vi "Slave - Interleaved Chs Dat Integrity.vi"() -> ()   [LabVIEW 2016]
uses:
  <vilib>/Utility/error.llb/DialogType.ctl
  <vilib>/pximc/Initialize Writer Session (DBL).vi
  <vilib>/pximc/Initialize Reader Session (DBL).vi
  <vilib>/pximc/Connect (DBL).vi
  <vilib>/pximc/Acquire Write Region (DBL).vi
  <vilib>/pximc/Acquire Read Region (DBL).vi
  <vilib>/pximc/nipximc.lvlib
  <resource>/objmgr/pximc.rc
panel:
  out "Writer Node 2":T1(graph)
  out "Writer Node 1":T1(graph)
  out "Stopped?":bool=TRUE
  in  "Stop Button":bool
  in  "#Writing Channels Slave 2":i32=2
  in  "#Reading Channels Slave 2":i32=4
  out "Reader Node 1":T1(graph)
  in  "#Reading Channels Slave 1":i32=4
  in  "#Writing Channels Slave 1":i32=2
  out "Reader Node 2":T1(graph)
  in  "Node 1 Reader Connection ID":u16=4
  in  "Reader Interface Node 2":tag="PXIMC2" caption="interface"
  in  "Node 2 Writer Connection ID":u16=3
  in  "Writer Interface Node 2":tag="PXIMC2" caption="interface"
  in  "Node 1 Writer Connection ID":u16=1
  in  "Node 1 Writer Interface":tag="PXIMC2" caption="interface"
  in  "Node 1 Reader Interface":tag="PXIMC2" caption="interface"
  in  "Buffer Size":u64=250000 caption="buffer size"
  in  "Connection Timeout (s)":dbl=60.0 caption="timeout in seconds (-1)"
  in  "Node 1 Reader Connection ID":u16=2
  # "Node 1"
  # "Node 2"
  # "Node 2 => Node 1"
  # "Node 1 => Node 2"
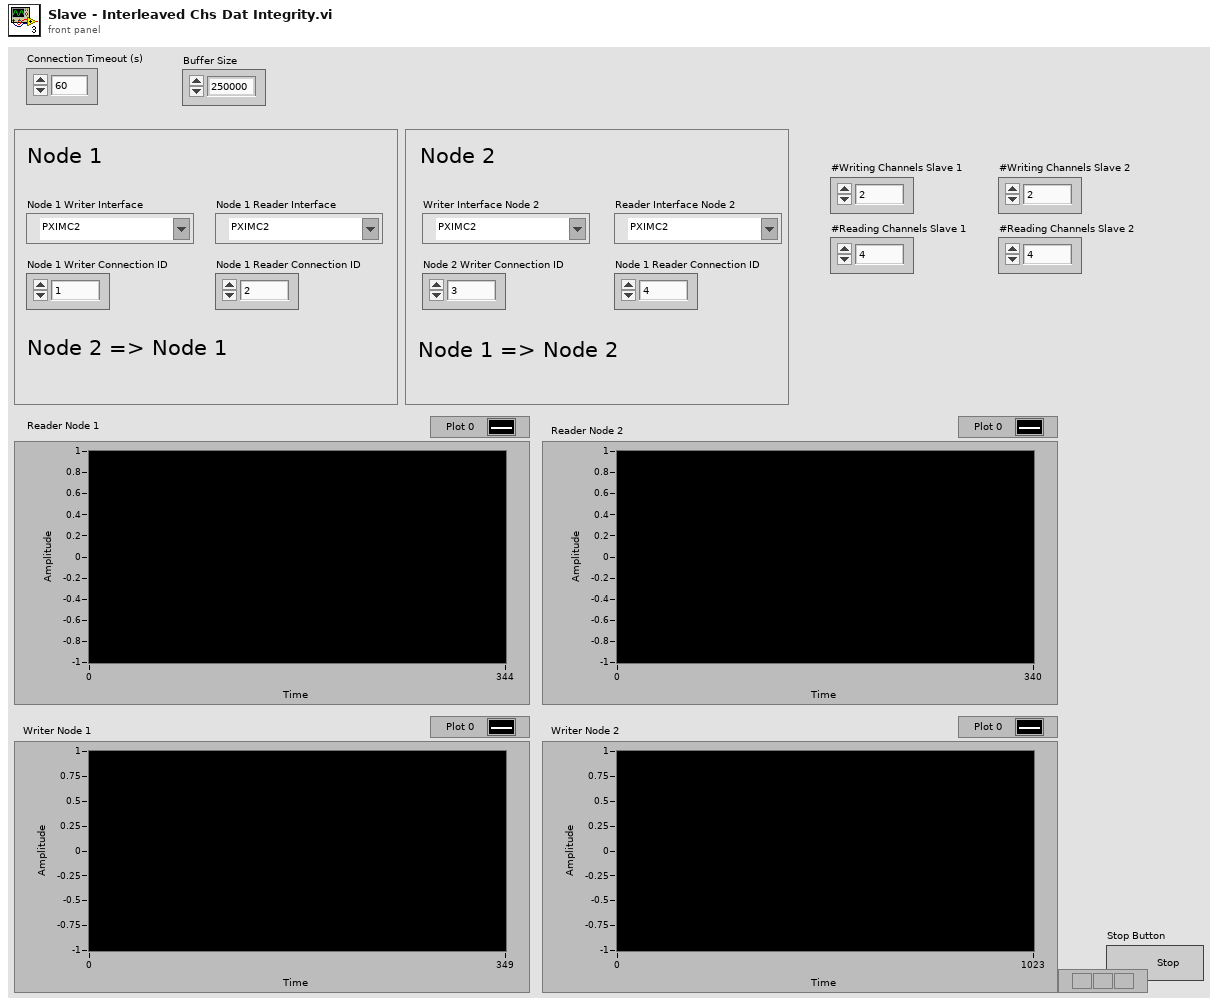
[diagram p1: front panel]
types:
  T1 = cluster{"[0]":dbl, "[1]":dbl, "[2]":dbl, "[3]":dbl, "[4]":dbl, "[5]":dbl, "[6]":dbl, "[7]":dbl, "[8]":dbl}
  T2 = typedef "DialogType.ctl" = u16
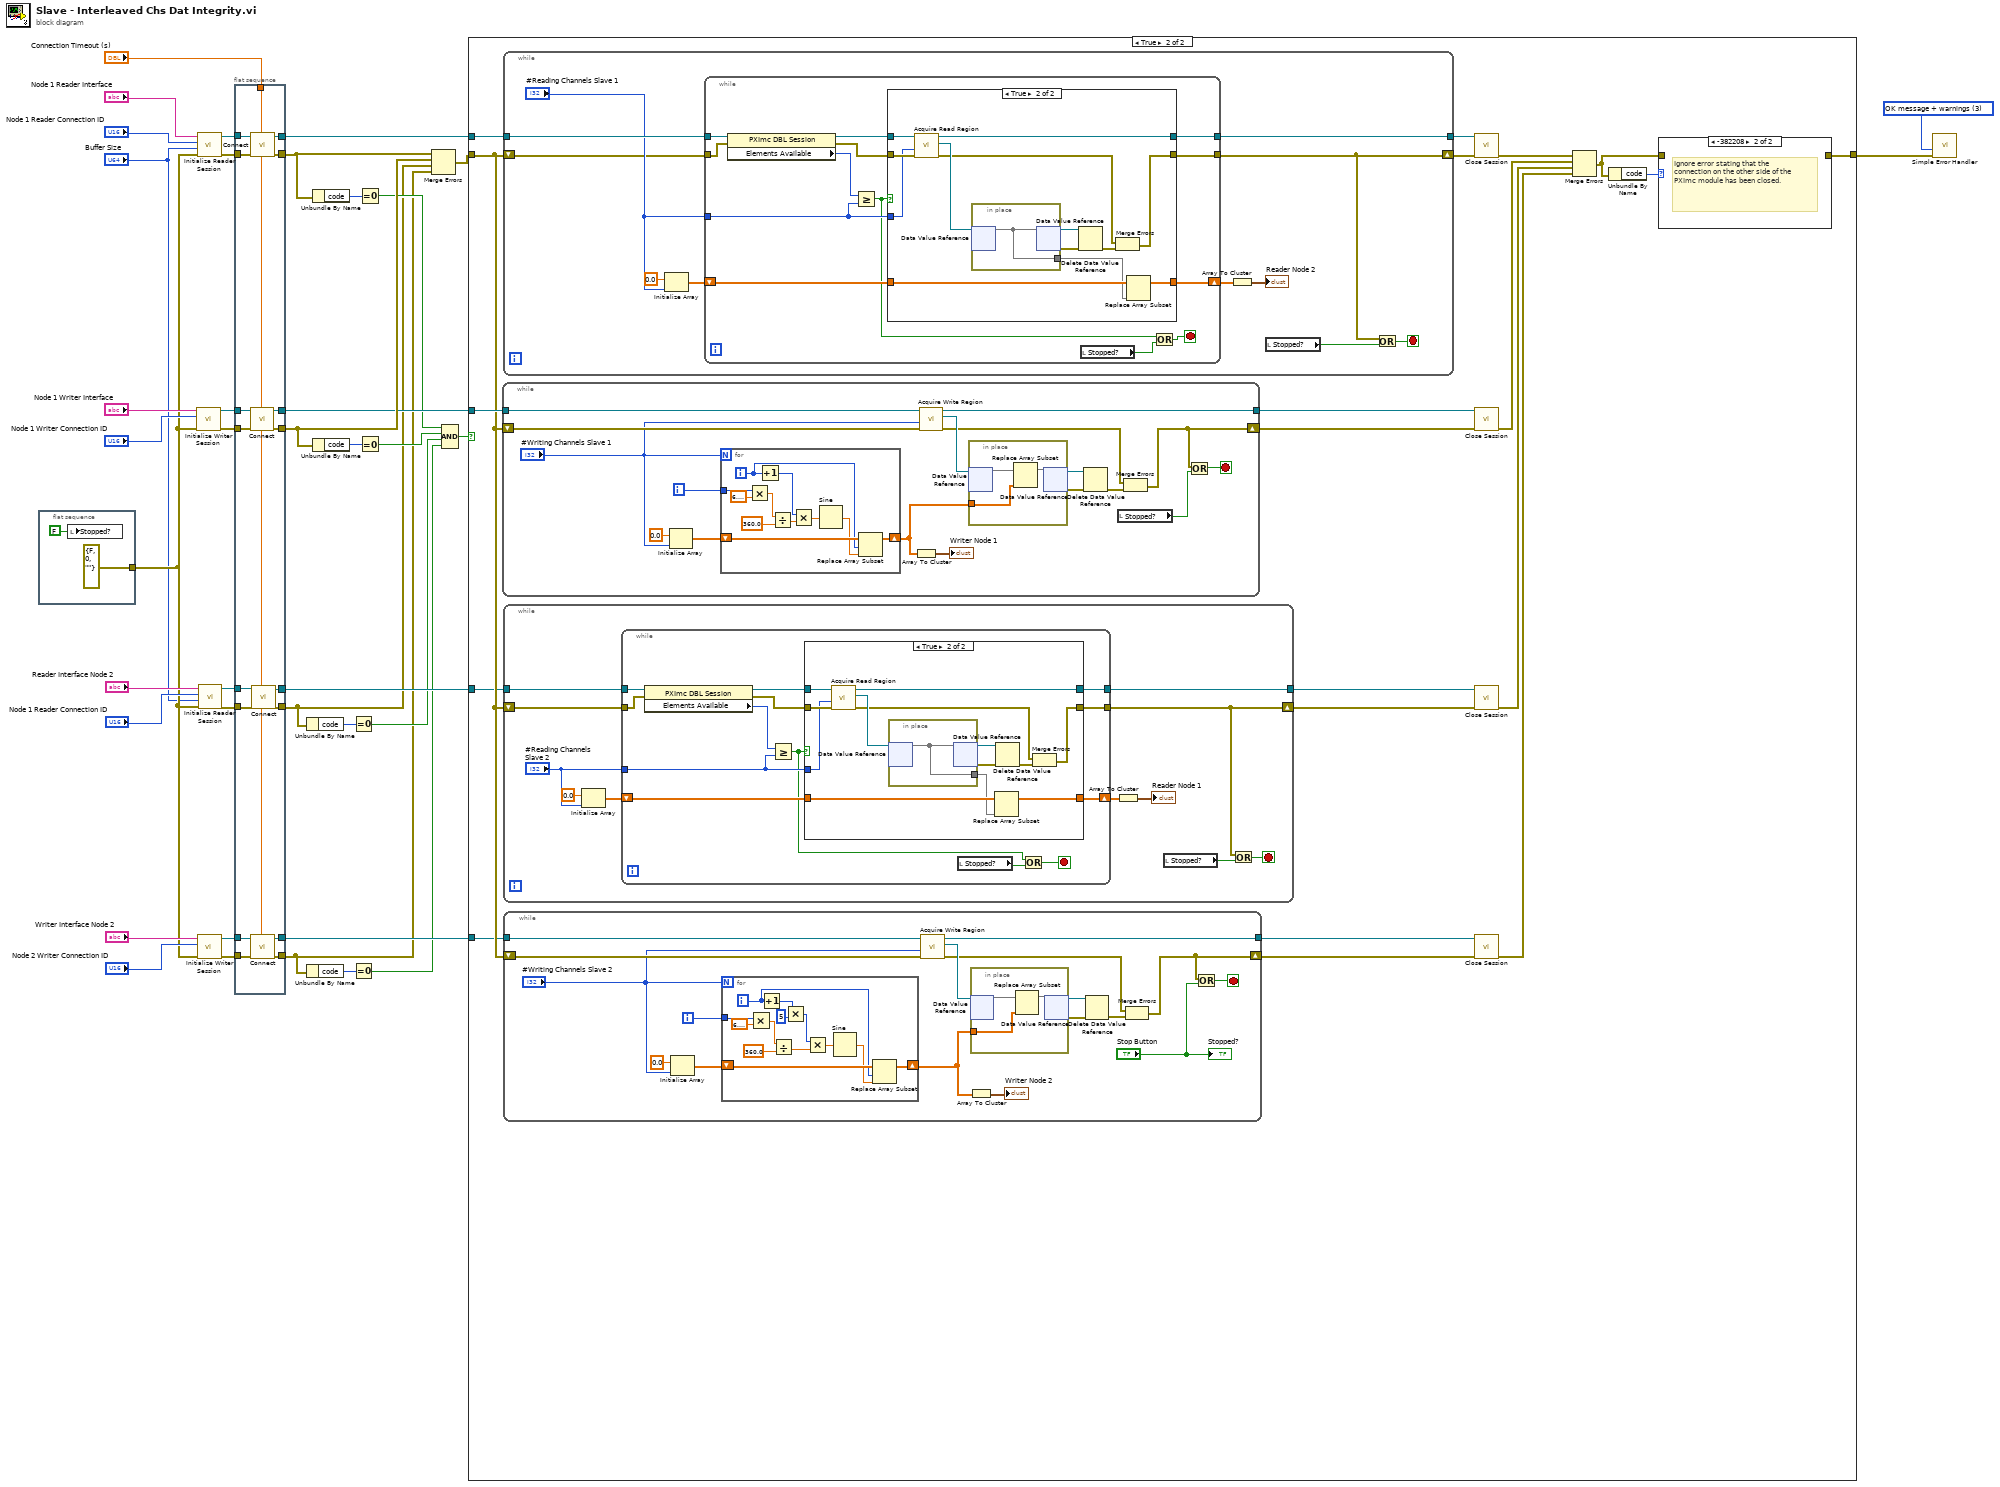
[diagram p0: block diagram]
diagram:
  w33 = T2 3 items=["no dialog", "OK message", "continue or stop message", "OK message + warnings", "continue/stop + warnings"] ("type of dialog (OK msg:1)")
  n1 = flat-sequence {
    tunnel: [errorcluster {"status"=FALSE, "code"=0, "source"=""} ("error constant")] -> w10
    frame #0 {
      n2 = local write "Stopped?"(FALSE ("Stopped?")) -> ()
    }
  }
  n3 = call-poly <vilib>:"Initialize Writer Session.vi"("error in (no error)"=w10, "connection id (1)"="Node 1 Writer Connection ID", "interface"="Node 1 Writer Interface") -> ("error out"=w31:errorcluster, "session out"=w30:refnum<k21>)  [unwired: 7 in]
  n4 = call-poly <vilib>:"Initialize Reader Session.vi"("error in (no error)"=w10, "buffer size"="Buffer Size", "writer's connection id (1)"="Node 1 Reader Connection ID", "interface"="Node 1 Reader Interface") -> ("error out"=w37:errorcluster, "session out"=w38:refnum<k21>)  [unwired: 6 in]
  n5 = call-poly <vilib>:"Initialize Writer Session.vi"("error in (no error)"=w10, "connection id (1)"="Node 2 Writer Connection ID", "interface"="Writer Interface Node 2") -> ("error out"=w17:errorcluster, "session out"=w18:refnum<k21>)  [unwired: 7 in]
  n6 = call-poly <vilib>:"Initialize Reader Session.vi"("error in (no error)"=w10, "buffer size"="Buffer Size", "writer's connection id (1)"="Node 1 Reader Connection ID", "interface"="Reader Interface Node 2") -> ("error out"=w13:errorcluster, "session out"=w12:refnum<k21>)  [unwired: 6 in]
  n7 = flat-sequence {
    tunnel: w38 -> [w58]
    tunnel: w37 -> [w57]
    tunnel: [w56] -> w36
    tunnel: w31 -> [w55]
    tunnel: w30 -> [w54]
    tunnel: [w53] -> w24
    tunnel: [w52] -> w23
    tunnel: "Connection Timeout (s)" -> [w42]
    tunnel: [w51] -> w21
    tunnel: [w50] -> w5
    tunnel: [w49] -> w1
    tunnel: [w48] -> w2
    tunnel: w18 -> [w47]
    tunnel: w17 -> [w46]
    tunnel: [w45] -> w6
    tunnel: w13 -> [w44]
    tunnel: w12 -> [w43]
    frame #0 {
      n8 = call-poly <vilib>:"Connect.vi"("timeout in seconds (-1)"=w42, "error in (no error)"=w55, "session in"=w54) -> ("error out"=w52:errorcluster, "session out"=w51:refnum<k21>)  [unwired: 7 in]
      n9 = call-poly <vilib>:"Connect.vi"("timeout in seconds (-1)"=w42, "error in (no error)"=w57, "session in"=w58) -> ("error out"=w53:errorcluster, "session out"=w56:refnum<k21>)  [unwired: 7 in]
      n10 = call-poly <vilib>:"Connect.vi"("timeout in seconds (-1)"=w42, "error in (no error)"=w46, "session in"=w47) -> ("error out"=w49:errorcluster, "session out"=w50:refnum<k21>)  [unwired: 7 in]
      n11 = call-poly <vilib>:"Connect.vi"("timeout in seconds (-1)"=w42, "error in (no error)"=w44, "session in"=w43) -> ("error out"=w48:errorcluster, "session out"=w45:refnum<k21>)  [unwired: 7 in]
    }
  }
  n12 = Unbundle By Name(w2) -> ("code"=w15:i32)
  n13 = Unbundle By Name(w1) -> ("code"=w20:i32)
  n14 = Unbundle By Name(w24) -> ("code"=w34:i32)
  n15 = Unbundle By Name(w23) -> ("code"=w28:i32)
  n16 = Equal To 0?(x=w15) -> (x = 0?=w4:bool)
  n17 = Equal To 0?(x=w20) -> (x = 0?=w3:bool)
  n18 = Equal To 0?(x=w34) -> (x = 0?=w8:bool)
  n19 = Equal To 0?(x=w28) -> (x = 0?=w26:bool)
  n20 = Merge Errors(w24, w23, w2, w1) -> (w25:errorcluster)
  n21 = Compound Arithmetic op=AND(w8, w26, w4, w3) -> (w27:bool)
  n22 = case shown="True" w27 {
    tunnel: w25 -> [w59 w73]
    tunnel: w36 -> [_ w77]
    tunnel: [w59 w79] -> w7
    tunnel: w21 -> [_ w75]
    tunnel: w6 -> [_ w72]
    tunnel: w5 -> [_ w71]
    frame False {
      # "The connection was not successful for some reason."
    }
    frame True {
      n23 = while {
        tunnel: w75 -> [w163]
        tunnel: [w162] -> w74
        shift-right: [w159] -> w67
        shift-left: w73 -> [w161]
        i -> [w154]
        stop <- w158 stop-if-true
        n24 = Initialize Array(0.0 ("element"), "#Writing Channels Slave 1") -> (w170:dbl[])
        n25 = for {
          N: "#Writing Channels Slave 1" -> [_]
          tunnel: w154 -> [w178]
          shift-right: [w176] -> w155
          shift-left: w170 -> [w177]
          i -> [w174]
          n26 = Multiply(x=w178, y=6.283185307179586) -> (x*y=w181:dbl)
          n27 = Increment(x=w174) -> (x+1=w179:i32)
          n28 = Divide(x=w181, y=360.0) -> (x/y=w183:dbl)
          n29 = Multiply(x=w179, y=w183) -> (x*y=w184:dbl)
          n30 = Sine(x=w184) -> (sin(x)=w175:dbl)
          n31 = Replace Array Subset(array=w177, new element=w175, index=w174) -> (w176:dbl[])
        }
        n32 = Array To Cluster(array=w155) -> (cluster=→"Writer Node 1":T1)
        n33 = call-poly <vilib>:"Acquire Write Region.vi"("error in (no error)"=w161, "number of elements"="#Writing Channels Slave 1", "session in"=w163) -> ("error out"=w164:errorcluster, "write region reference"=w165:refnum<data-value>, "session out"=w162:refnum<k21>)  [unwired: 5 in, 1 out]
        n34 = in-place {
          in-place-border: w155 -> [w171]
          n35 = in-place-dvr #1(w165) -> (w173:dbl[])  [unwired: 1 out]
          n36 = Replace Array Subset(array=w173, new element=w171) -> (w172:dbl[])  [unwired: 1 in]
          n37 = in-place-dvr #1(w172) -> (w166:refnum<data-value>, w168:errorcluster)
        }
        n38 = Delete Data Value Reference(data value reference=w166, error in=w168) -> (error out=w167:errorcluster)  [unwired: 1 out]
        n39 = local read "Stopped?"() -> (w157:bool)
        n40 = Merge Errors(w164, w167) -> (w159:errorcluster)
        n41 = Or(x=w159, y=w157) -> (x .or. y?=w158:bool)
      }
      n42 = while {
        tunnel: [w189] -> w76
        shift-right: [w188] -> w68
        shift-left: w73 -> [w186]
        tunnel: w77 -> [w193]
        stop <- w195 stop-if-true
        n43 = Initialize Array(0.0 ("element"), "#Reading Channels Slave 1") -> (w192:dbl[])
        n44 = while {
          tunnel: w193 -> [w207]
          tunnel: w186 -> [w204]
          tunnel: [w208] -> w188
          tunnel: "#Reading Channels Slave 1" -> [w200]
          shift-right: [w201] -> w187
          shift-left: w192 -> [w202]
          tunnel: [w199] -> w189
          stop <- w196 stop-if-true
          n45 = property class="PXImc DBL Session"(reference=w207, error in=w204) -> (reference out=w205:refnum<k21>, error out=w203:errorcluster, "Elements Available"=w206:u64)
          n46 = Greater Or Equal?(x=w206, y=w200) -> (x >= y?=w198:bool)
          n47 = case shown="True" w198 {
            tunnel: w203 -> [w211 w223]
            tunnel: [w211 w217] -> w208
            tunnel: w205 -> [w209 w222]
            tunnel: w202 -> [w210 w216]
            tunnel: [w210 w214] -> w201
            tunnel: w200 -> [_ w213]
            tunnel: [w209 w212] -> w199
            frame False {
            }
            frame True {
              n48 = call-poly <vilib>:"Acquire Read Region.vi"("error in (no error)"=w223, "number of elements"=w213, "session in"=w222) -> ("error out"=w218:errorcluster, "read region reference"=w224:refnum<data-value>, "session out"=w212:refnum<k21>)  [unwired: 5 in, 1 out]
              n49 = in-place {
                in-place-border: [w225] -> w215
                n50 = in-place-dvr #2(w224) -> (w225:dbl[])  [unwired: 1 out]
                n51 = in-place-dvr #2(w225) -> (w221:refnum<data-value>, w220:errorcluster)
              }
              n52 = Delete Data Value Reference(data value reference=w221, error in=w220) -> (error out=w219:errorcluster)  [unwired: 1 out]
              n53 = Merge Errors(w218, w219) -> (w217:errorcluster)
              n54 = Replace Array Subset(array=w216, new element=w215) -> (w214:dbl[])  [unwired: 1 in]
            }
          }
          n55 = local read "Stopped?"() -> (w197:bool)
          n56 = Or(x=w198, y=w197) -> (x .or. y?=w196:bool)
        }
        n57 = Array To Cluster(array=w187) -> (cluster=→"Reader Node 2":T1)
        n58 = local read "Stopped?"() -> (w185:bool)
        n59 = Or(x=w188, y=w185) -> (x .or. y?=w195:bool)
      }
      n60 = while {
        tunnel: [w117] -> w69
        shift-right: [w114] -> w66
        shift-left: w73 -> [w115]
        tunnel: w72 -> [w121]
        stop <- w123 stop-if-true
        n61 = Initialize Array(0.0 ("element"), "#Reading Channels Slave 2") -> (w120:dbl[])
        n62 = while {
          tunnel: w121 -> [w135]
          tunnel: w115 -> [w132]
          tunnel: [w136] -> w114
          tunnel: "#Reading Channels Slave 2" -> [w128]
          shift-right: [w129] -> w116
          shift-left: w120 -> [w130]
          tunnel: [w127] -> w117
          stop <- w124 stop-if-true
          n63 = property class="PXImc DBL Session"(reference=w135, error in=w132) -> (reference out=w133:refnum<k21>, error out=w131:errorcluster, "Elements Available"=w134:u64)
          n64 = Greater Or Equal?(x=w134, y=w128) -> (x >= y?=w125:bool)
          n65 = case shown="True" w125 {
            tunnel: w131 -> [w139 w151]
            tunnel: [w139 w145] -> w136
            tunnel: w133 -> [w137 w150]
            tunnel: w130 -> [w138 w144]
            tunnel: [w138 w142] -> w129
            tunnel: w128 -> [_ w141]
            tunnel: [w137 w140] -> w127
            frame False {
            }
            frame True {
              n66 = call-poly <vilib>:"Acquire Read Region.vi"("error in (no error)"=w151, "number of elements"=w141, "session in"=w150) -> ("error out"=w146:errorcluster, "read region reference"=w152:refnum<data-value>, "session out"=w140:refnum<k21>)  [unwired: 5 in, 1 out]
              n67 = in-place {
                in-place-border: [w153] -> w143
                n68 = in-place-dvr #3(w152) -> (w153:dbl[])  [unwired: 1 out]
                n69 = in-place-dvr #3(w153) -> (w149:refnum<data-value>, w148:errorcluster)
              }
              n70 = Replace Array Subset(array=w144, new element=w143) -> (w142:dbl[])  [unwired: 1 in]
              n71 = Delete Data Value Reference(data value reference=w149, error in=w148) -> (error out=w147:errorcluster)  [unwired: 1 out]
              n72 = Merge Errors(w146, w147) -> (w145:errorcluster)
            }
          }
          n73 = local read "Stopped?"() -> (w126:bool)
          n74 = Or(x=w125, y=w126) -> (x .or. y?=w124:bool)
        }
        n75 = Array To Cluster(array=w116) -> (cluster=→"Reader Node 1":T1)
        n76 = local read "Stopped?"() -> (w113:bool)
        n77 = Or(x=w114, y=w113) -> (x .or. y?=w123:bool)
      }
      n78 = while {
        tunnel: w71 -> [w89]
        tunnel: [w88] -> w70
        shift-right: [w85] -> w65
        shift-left: w73 -> [w87]
        i -> [w82]
        stop <- w84 stop-if-true
        n79 = Initialize Array(0.0 ("element"), "#Writing Channels Slave 2") -> (w96:dbl[])
        n80 = for {
          N: "#Writing Channels Slave 2" -> [_]
          tunnel: w82 -> [w107]
          shift-right: [w105] -> w80
          shift-left: w96 -> [w106]
          i -> [w103]
          n81 = Multiply(x=w107, y=6.283185307179586) -> (x*y=w109:dbl)
          n82 = Increment(x=w103) -> (x+1=w102:i32)
          n83 = Divide(x=w109, y=360.0) -> (x/y=w111:dbl)
          n84 = Multiply(x=w102, y=5) -> (x*y=w100:i32)
          n85 = Multiply(x=w100, y=w111) -> (x*y=w112:dbl)
          n86 = Sine(x=w112) -> (sin(x)=w104:dbl)
          n87 = Replace Array Subset(array=w106, new element=w104, index=w103) -> (w105:dbl[])
        }
        n88 = call-poly <vilib>:"Acquire Write Region.vi"("error in (no error)"=w87, "number of elements"="#Writing Channels Slave 2", "session in"=w89) -> ("error out"=w90:errorcluster, "write region reference"=w91:refnum<data-value>, "session out"=w88:refnum<k21>)  [unwired: 5 in, 1 out]
        n89 = Array To Cluster(array=w80) -> (cluster=→"Writer Node 2":T1)
        n90 = in-place {
          in-place-border: w80 -> [w97]
          n91 = in-place-dvr #4(w91) -> (w99:dbl[])  [unwired: 1 out]
          n92 = Replace Array Subset(array=w99, new element=w97) -> (w98:dbl[])  [unwired: 1 in]
          n93 = in-place-dvr #4(w98) -> (w92:refnum<data-value>, w94:errorcluster)
        }
        n94 = Delete Data Value Reference(data value reference=w92, error in=w94) -> (error out=w93:errorcluster)  [unwired: 1 out]
        n95 = Merge Errors(w90, w93) -> (w85:errorcluster)
        n96 = Or(x=w85, y="Stop Button") -> (x .or. y?=w84:bool)
        "Stopped?" <- "Stop Button"
      }
      n97 = call <vilib>:"Close Session.vi"("error in (no error)"=w68, "session in"=w76) -> ("error out"=w64:errorcluster)  [unwired: 9 in]
      n98 = call <vilib>:"Close Session.vi"("error in (no error)"=w67, "session in"=w74) -> ("error out"=w63:errorcluster)  [unwired: 9 in]
      n99 = call <vilib>:"Close Session.vi"("error in (no error)"=w66, "session in"=w69) -> ("error out"=w62:errorcluster)  [unwired: 9 in]
      n100 = call <vilib>:"Close Session.vi"("error in (no error)"=w65, "session in"=w70) -> ("error out"=w61:errorcluster)  [unwired: 9 in]
      n101 = Merge Errors(w64, w63, w62, w61) -> (w60:errorcluster)
      n102 = Unbundle By Name(w60) -> ("code"=w78:i32)
      n103 = case shown="-382208" w78 {
        tunnel: w60 -> [w226 _]
        tunnel: [w226 _] -> w79
        frame 0, Default {
        }
        frame -382208 {
          # "Ignore error stating that the connection on the other side of the PXImc module has been closed."
        }
      }
    }
  }
  n104 = call <vilib>:"Simple Error Handler.vi"("type of dialog (OK msg:1)"=w33, "error in (no error)"=w7) -> ()  [unwired: 3 in, 5 out]
